vi "AI0-1.vi"() -> ()   [LabVIEW 2012]
uses:
  <vilib>/rvi/eio/common/nirviEmuTemplateMethod_errors.vi
  <vilib>/eio/EIONode/EIONode.xnode
panel:
  out "Connector0/AI1":i16
  out "Connector0/AI0":i16
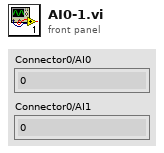
[diagram p1: front panel]
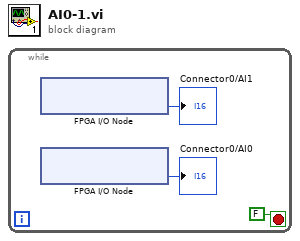
[diagram p0: block diagram]
diagram:
  n1 = while {
    stop <- FALSE stop-if-true
    n2 = xnode "FPGA I/O Node"() -> ("Connector0/AI1"=→"Connector0/AI1":i16)  [unwired: 1 in, 1 out]
    n3 = xnode "FPGA I/O Node"() -> ("Connector0/AI0"=→"Connector0/AI0":i16)  [unwired: 1 in, 1 out]
  }
